vi "autoExposureOn.vi"(8 "error in (no error)":errorcluster, 11 "Camera in":refnum<class "Camera.lvclass">) -> (0 "error out":errorcluster, 3 "Camera out":refnum<class "Camera.lvclass">)   [LabVIEW 2019, in "Camera.lvclass"]
doc: "Enables auto-exposure mode for recording."
uses:
  Camera.lvclass
  Camera.lvclass/Camera.ctl
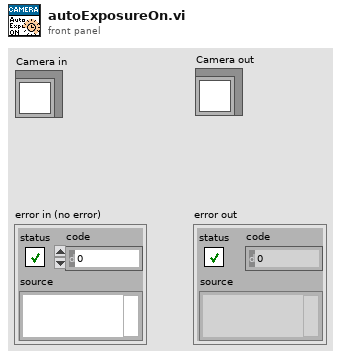
[diagram p1: front panel]
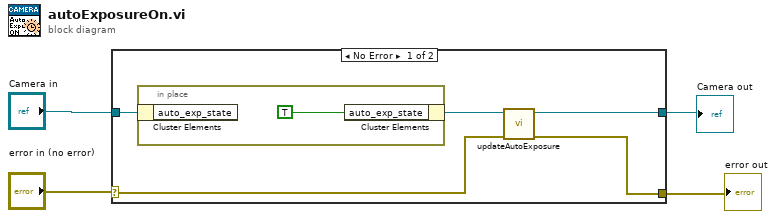
[diagram p0: block diagram]
diagram:
  n1 = case shown="No Error" "error in (no error)" {
    selector: "error in (no error)" -> [w6 w12]
    tunnel: [w5 w12] -> w3
    tunnel: "Camera in" -> [w9 w11]
    tunnel: [w7 w11] -> w1
    frame No Error {
      n2 = in-place {
        n3 = in-place-cluster #1(w9) -> ()  [unwired: 1 out]
        n4 = in-place-cluster #1("auto_exp_state"=TRUE ("AutoExposureState")) -> (w8:refnum<class "Camera.lvclass">)
      }
      n5 = call "updateAutoExposure.vi"("error in (no error)"=w6, "Camera in"=w8) -> ("error out"=w5:errorcluster, "Camera out"=w7:refnum<class "Camera.lvclass">)  [unwired: 8 in]
    }
    frame Error {
    }
  }
  "Camera out" <- w1
  "error out" <- w3
